vi "Read 2 Traces.vi"(8 "error in (no error)":errorcluster, 11 "VISA Resource Name":refnum<visa-resource-name>) -> (0 "error out":errorcluster, 1 "Y":dbl format="%.4e", 2 "X":dbl format="%.4e", 3 "VISA Resource Name Out":refnum<visa-resource-name>, 4 "theta":dbl, 5 "r":dbl)   [LabVIEW 2015]
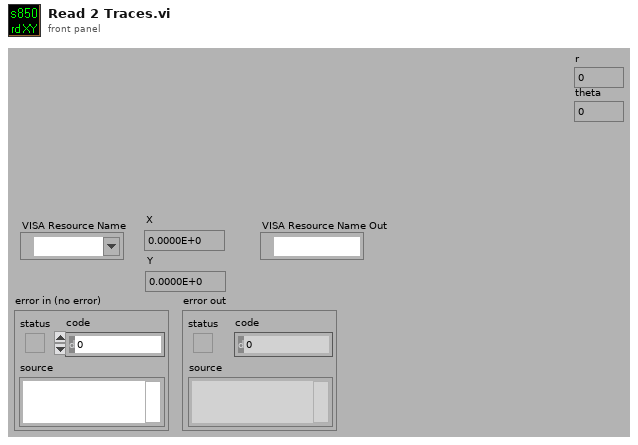
[diagram p1: front panel]
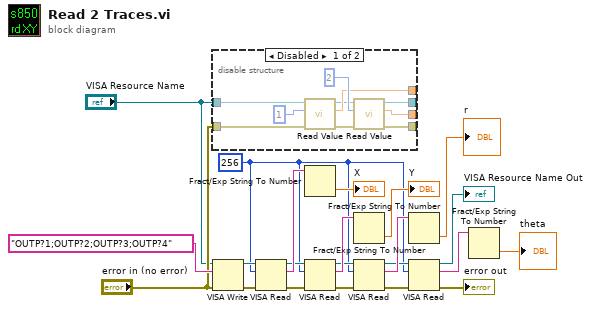
[diagram p0: block diagram]
diagram:
  w1 = u32 256 ("byte count")
  n1 = disable-structure shown="Disabled" {
    disable-tunnel: [w32 _] -> _
    disable-tunnel: "error in (no error)" -> [w29 _]
    disable-tunnel: [w28 _] -> _
    disable-tunnel: [w27 _] -> _
    disable-tunnel: "VISA Resource Name" -> [w25 _]
    disable-tunnel: [w23 _] -> _
    frame Disabled {
      n2 = call "Read Value.vi"("error in (no error)"=w29, "Trace"=i16 1, "VISA Resource Name"=w25) -> ("error out"=w30:errorcluster, "Value"=w28:dbl, "VISA Resource Name Out"=w24:refnum<visa-resource-name>)  [unwired: 6 out]
      n3 = call "Read Value.vi"("error in (no error)"=w30, "Trace"=i16 2, "VISA Resource Name"=w24) -> ("error out"=w27:errorcluster, "Value"=w32:dbl, "VISA Resource Name Out"=w23:refnum<visa-resource-name>)  [unwired: 6 out]
    }
    frame Enabled {
    }
  }
  n4 = VISA Write(VISA resource name="VISA Resource Name", write buffer="OUTP?1;OUTP?2;OUTP?3;OUTP?4", error in (no error)="error in (no error)") -> (VISA resource name out=w21:refnum<visa-resource-name>, error out=w22:errorcluster)  [unwired: 1 out]
  n5 = VISA Read(VISA resource name=w21, byte count=w1, error in (no error)=w22) -> (VISA resource name out=w12:refnum<visa-resource-name>, read buffer=w19:string, error out=w13:errorcluster)  [unwired: 1 out]
  n6 = Fract/Exp String To Number(string=w19) -> (number=→"X":dbl)  [unwired: 4 out]
  n7 = VISA Read(VISA resource name=w12, byte count=w1, error in (no error)=w13) -> (VISA resource name out=w8:refnum<visa-resource-name>, read buffer=w18:string, error out=w5:errorcluster)  [unwired: 1 out]
  n8 = Fract/Exp String To Number(string=w18) -> (number=→"Y":dbl)  [unwired: 4 out]
  n9 = VISA Read(VISA resource name=w8, byte count=w1, error in (no error)=w5) -> (VISA resource name out=w9:refnum<visa-resource-name>, read buffer=w11:string, error out=w6:errorcluster)  [unwired: 1 out]
  n10 = Fract/Exp String To Number(string=w11) -> (number=→"r":dbl)  [unwired: 4 out]
  n11 = VISA Read(VISA resource name=w9, byte count=w1, error in (no error)=w6) -> (VISA resource name out=→"VISA Resource Name Out":refnum<visa-resource-name>, read buffer=w10:string, error out=→"error out":errorcluster)  [unwired: 1 out]
  n12 = Fract/Exp String To Number(string=w10) -> (number=→"theta":dbl)  [unwired: 4 out]
